vi "ConvertDataListToArray.vi"(11 "Data List":string) -> (3 "Values":dbl[](array[numeric]))   [LabVIEW 2010, in "Keithley-6482-Visa.lvlib"]
uses:
  <instrlib>/lib-labview-8.6-export/Keithley-6482-Visa.lvlib
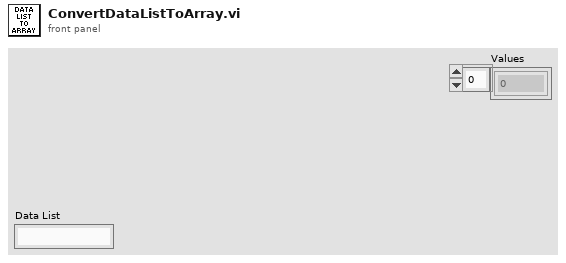
[diagram p1: front panel]
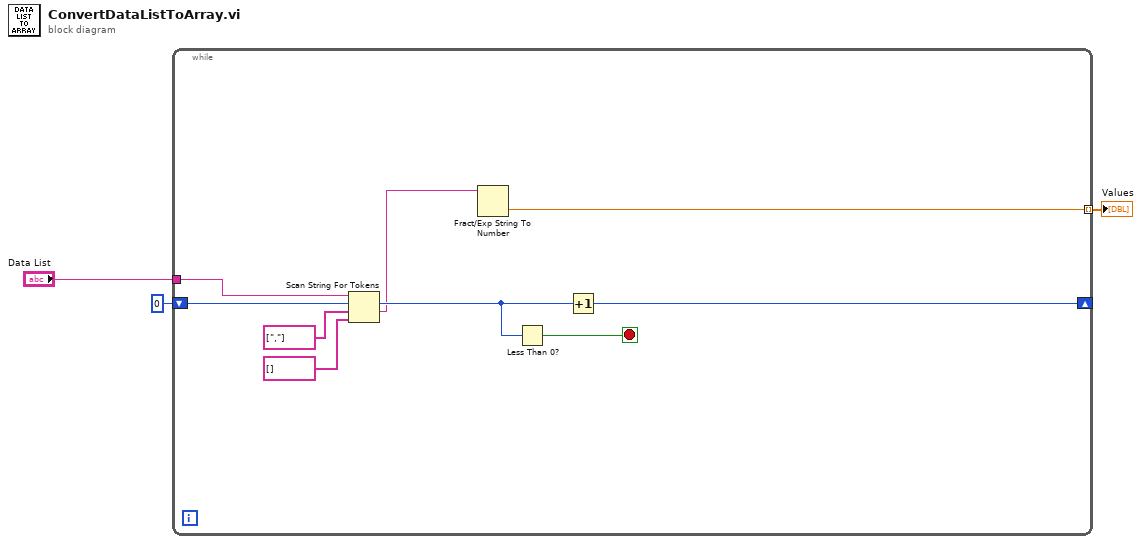
[diagram p0: block diagram]
diagram:
  n1 = while {
    shift-right: [w6] -> _
    shift-left: 0 ("offset past token") -> [w12]
    tunnel: "Data List" -> [w9]
    tunnel: [w4] -> w1 mode=indexing
    stop <- w8 stop-if-true
    n2 = Scan String For Tokens(6:string[] [] ("delimiters (\\s,\\t,\\r,\\n)"), 7:string[] [","] ("delimiters (\\s,\\t,\\r,\\n)"), 8:w12, 9:w9) -> (1:w5:string, 2:w7:i32)  [unwired: 2 in, 2 out]
    n3 = Fract/Exp String To Number(string=w5) -> (number=w4:dbl)  [unwired: 3 in, 1 out]
    n4 = Less Than 0?(x=w7) -> (x < 0?=w8:bool)
    n5 = Increment(x=w7) -> (x+1=w6:i32)
  }
  "Values" <- w1
